vi "Utility Check for More to Read.vi"(8 "error in (no error)":errorcluster, 11 "VISA Refnum in":refnum<visa-resource-name>) -> (0 "error out (unchanged)":errorcluster, 2 "More to read?":bool, 3 "VISA Refnum out":refnum<visa-resource-name>)   [LabVIEW 2020, in "ChromTech Series III Pump.lvlib"]
doc: "Checks the bytes at port on an error for the given VISA resource to confirm if all bytes have been read or if there is more to read."
uses:
  <instrlib>/ChromTech Series III Pump/ChromTech Series III Pump.lvlib
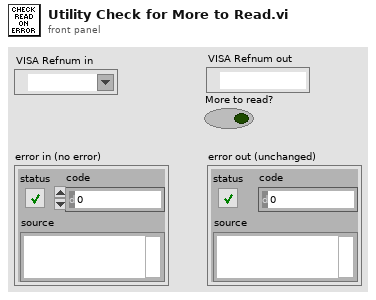
[diagram p1: front panel]
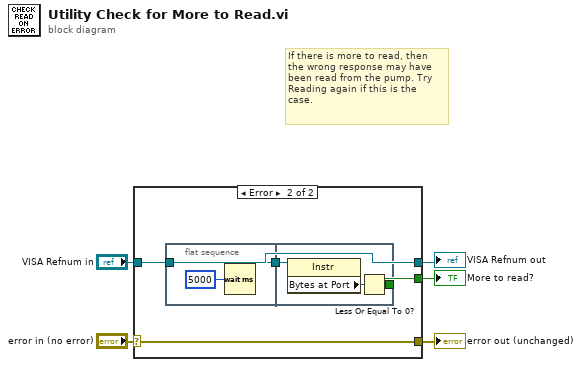
[diagram p0: block diagram]
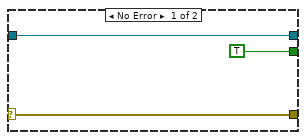
[diagram p2: hidden frame]
diagram:
  # "If there is more to read, then\nthe wrong response may have\nbeen read from the pump. Try\nReading again if this is the\ncase."
  n1 = case shown="Error" "error in (no error)" {
    selector: "error in (no error)" -> [w7 w11]
    tunnel: "VISA Refnum in" -> [w6 w10]
    tunnel: [TRUE w12] -> w3
    tunnel: [w7 w11] -> w2
    tunnel: [w6 w10] -> w1
    frame No Error {
    }
    frame Error {
      n2 = flat-sequence {
        tunnel: w10 -> [w14]
        tunnel: [w14] -> w9
        tunnel: [w16] -> w12
        tunnel: w9 -> [w15]
        frame #0 {
          n3 = Wait (ms)(milliseconds to wait=u32 5000) -> ()  [unwired: 1 out]
        }
        frame #1 {
          n4 = property class="Instr"(reference=w15) -> ("Bytes at Port"=w17:u32)  [unwired: 1 in, 2 out]
          n5 = Less Or Equal To 0?(x=w17) -> (x <= 0?=w16:bool)
        }
      }
    }
  }
  "More to read?" <- w3
  "error out (unchanged)" <- w2
  "VISA Refnum out" <- w1
